vi "bits2image.vi"(1 "Bitstream Input":u8[][](array[numeric])) -> (0 "new picture":picture caption="新图片")   [LabVIEW 2019]
uses:
  <vilib>/picture/picture.llb/Draw True-Color Pixmap.vi
panel:
  out "2D JPG Array":u32[][](array[numeric])
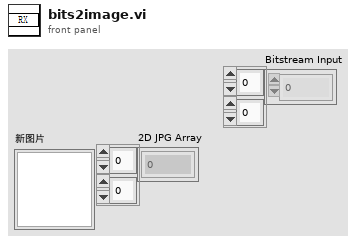
[diagram p1: front panel]
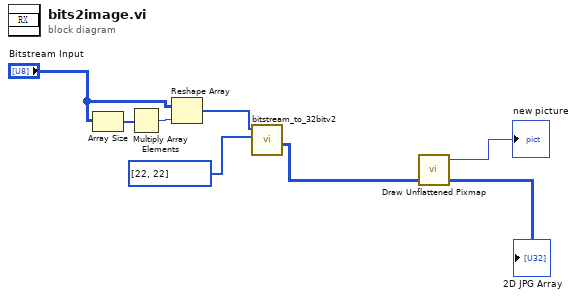
[diagram p0: block diagram]
diagram:
  n1 = Array Size(array="Bitstream Input") -> (size(s)=w3:i32[])
  n2 = Multiply Array Elements(1:w3) -> (0:w4:i32)
  n3 = Reshape Array "Reshape Array"("Bitstream Input", w4) -> (w1:u8[])
  n4 = call "bitstream_to_32bitv2.vi"("JPG Size"=i32[] [22, 22], "Bitstream Input"=w1) -> ("2D JPG Array"=w7:u32[][])  [unwired: 8 in, 1 out]
  "2D JPG Array" <- w7
  n5 = call-poly <vilib>:"Draw Unflattened Pixmap.vi"("data (RGB format)"=w7) -> ("new picture"=→"new picture":picture)  [unwired: 8 in]
